vi "Graphics-LTWH to LTRB (clusters).vi"(4 "LTWH":T1) -> (1 "LTRB":T2)   [LabVIEW 2020]
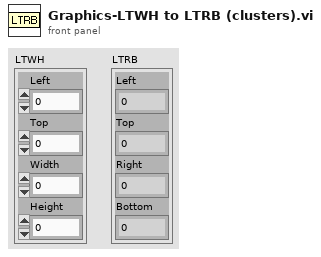
[diagram p1: front panel]
types:
  T1 = cluster{"Left":i16, "Top":i16, "Width":i16, "Height":i16}
  T2 = cluster{"Left":i16, "Top":i16, "Right":i16, "Bottom":i16}
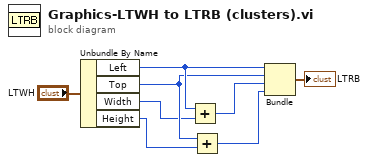
[diagram p0: block diagram]
diagram:
  n1 = Unbundle By Name("LTWH") -> ("Left"=w4:i16, "Top"=w3:i16, "Width"=w2:i16, "Height"=w1:i16)
  n2 = Add(x=w4, y=w2) -> (x+y=w8:i16)
  n3 = Add(x=w3, y=w1) -> (x+y=w7:i16)
  n4 = Bundle("Left"=w4, "Top"=w3, w8, w7) -> (→"LTRB":cluster{"Left":i16, "Top":i16, i16, i16})  [unwired: 1 in]
